vi "Write SwitchDMM Channel.vi"(8 "error in (no error)":errorcluster, 10 "SwitchDMM Channel":T1={"Switch"="V"}, 11 "SwitchDMM Channel configuration":refnum<class "SwitchDMM Channel configuration.lvclass">) -> (0 "error out":errorcluster, 3 "SwitchDMM Channel configuration out":refnum<class "SwitchDMM Channel configuration.lvclass">)   [LabVIEW 2025, in "SwitchDMM Channel configuration.lvclass"]
uses:
  SwitchDMM Channel configuration.lvclass
  SwitchDMM Channel.ctl
  SwitchDMM Channel configuration.lvclass/SwitchDMM Channel configuration.ctl
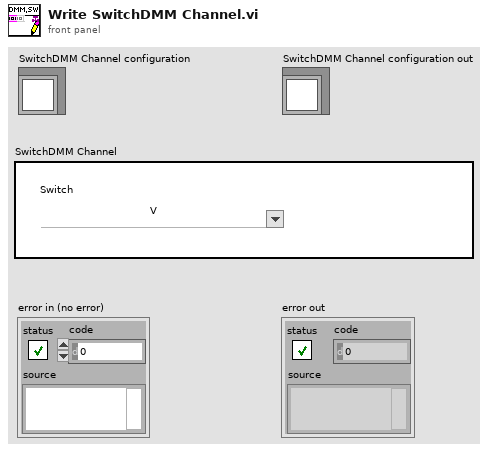
[diagram p1: front panel]
types:
  T1 = typedef "SwitchDMM Channel configuration.lvclass/SwitchDMM Channel.ctl" = cluster{"Switch":string}
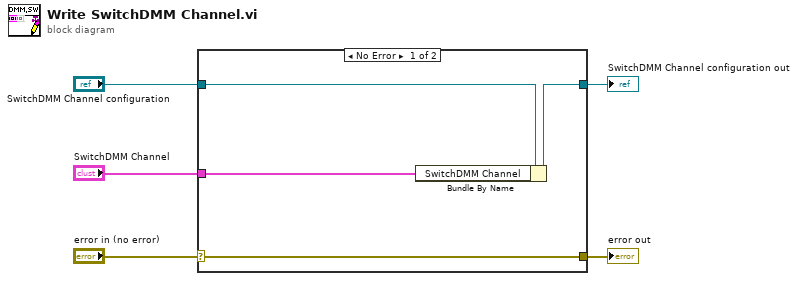
[diagram p0: block diagram]
diagram:
  n1 = case shown="No Error" "error in (no error)" {
    selector: "error in (no error)" -> [w9 w10]
    tunnel: [w9 w10] -> w4
    tunnel: [w7 w11] -> w3
    tunnel: "SwitchDMM Channel configuration" -> [w8 w11]
    tunnel: "SwitchDMM Channel" -> [w6 _]
    frame No Error {
      n2 = Bundle By Name(cluster=w8, "SwitchDMM Channel"=w6) -> (w7:refnum<class "SwitchDMM Channel configuration.lvclass">)
    }
    frame Error {
    }
  }
  "error out" <- w4
  "SwitchDMM Channel configuration out" <- w3
